vi "Interpolation_Box.vi"(6 "Current step":i32, 10 "sweep parameters":T1) -> (0 "completion":dbl, 2 "Value":dbl, 4 "Finished":bool)   [LabVIEW 2009]
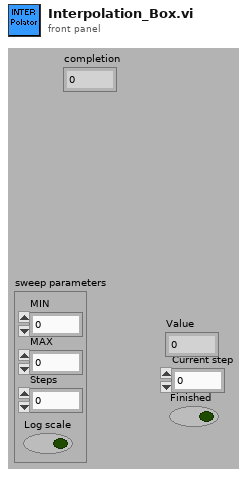
[diagram p1: front panel]
types:
  T1 = cluster{"MIN":dbl, "MAX":dbl, "Steps":dbl, "Log scale":bool}
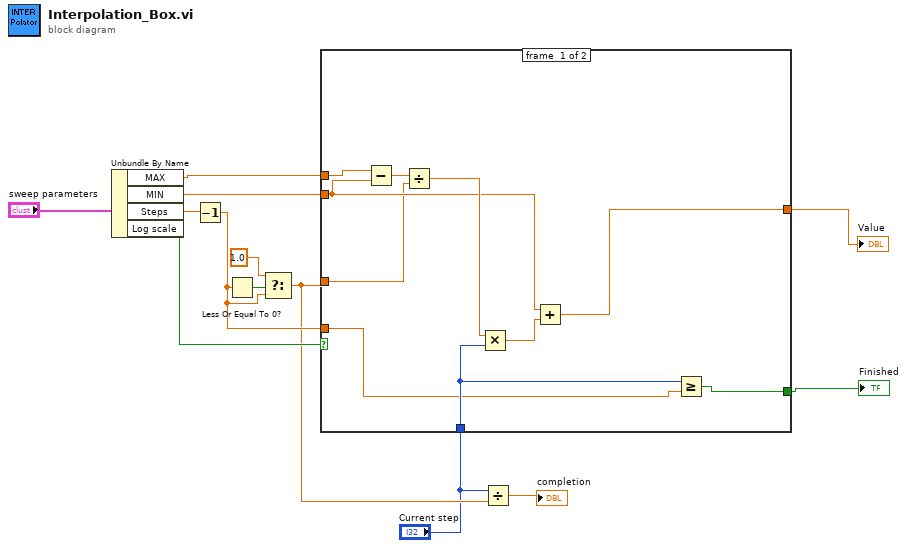
[diagram p0: block diagram]
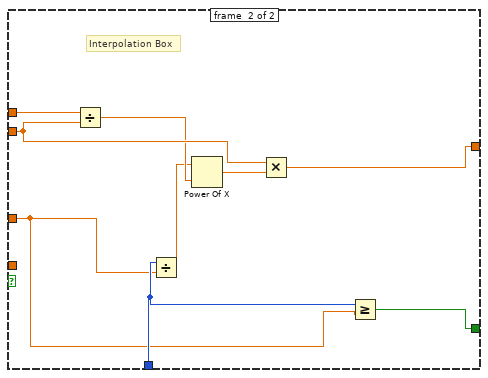
[diagram p2: hidden frame]
diagram:
  n1 = Unbundle By Name("sweep parameters") -> ("MAX"=w9:dbl, "MIN"=w8:dbl, "Steps"=w7:dbl, "Log scale"=w11:bool)
  n2 = Decrement(x=w7) -> (x-1=w4:dbl)
  n3 = Less Or Equal To 0?(x=w4) -> (x <= 0?=w6:bool)
  n4 = Select(t=1.0, s=w6, f=w4) -> (s? t:f=w3:dbl)
  n5 = case shown="False" w11 {
    tunnel: w9 -> [w20 w26]
    tunnel: w8 -> [w21 w32]
    tunnel: w3 -> [w14 w24]
    tunnel: "Current step" -> [w17 w27]
    tunnel: [w18 w31] -> w12
    tunnel: [w16 w25] -> w13
    tunnel: w4 -> [w15 _]
    frame #0 {
      n6 = Subtract(x=w20, y=w21) -> (x-y=w23:dbl)
      n7 = Divide(x=w23, y=w14) -> (x/y=w22:dbl)
      n8 = Multiply(x=w22, y=w17) -> (x*y=w19:dbl)
      n9 = Add(x=w21, y=w19) -> (x+y=w18:dbl)
      n10 = Greater Or Equal?(x=w17, y=w15) -> (x >= y?=w16:bool)
    }
    frame #1 {
      # "Interpolation Box"
      n11 = Divide(x=w26, y=w32) -> (x/y=w30:dbl)
      n12 = Divide(x=w27, y=w24) -> (x/y=w29:dbl)
      n13 = Power Of X(1:w30, 2:w29) -> (0:w28:dbl)
      n14 = Multiply(x=w32, y=w28) -> (x*y=w31:dbl)
      n15 = Greater Or Equal?(x=w27, y=w24) -> (x >= y?=w25:bool)
    }
  }
  "Finished" <- w13
  "Value" <- w12
  n16 = Divide(x="Current step", y=w3) -> (x/y=→"completion":dbl)
